vi "Parse-attributes.vi"(8 "error in (no error)":errorcluster, 10 "String in":string, 11 "Set in":refnum<class "Set.lvclass">) -> (0 "error out":errorcluster, 1 "Valid attributes?":bool, 2 "Remaining string":string, 3 "Set out":refnum<class "Set.lvclass">, 4 "Remaining content?":bool)   [LabVIEW 2013, in "HardwareCharacterization.lvlib" / "Set.lvclass"]
uses:
  Set.lvclass
  Attribute-XML/Attributes.ctl
  Attribute-XML/ID/Attribute-ID.ctl
  Attribute-XML/Attribute-XML.lvclass
  Attribute-XML/ID/FieldOffset/FieldOffset.lvclass
  Attribute-XML/ID/TransformEnable/TransformEnable.lvclass
  Attribute-XML/ID/Transform/Transform.lvclass
  Attribute-XML/ID/Units/Units.lvclass
  Attribute-XML/ID/XYCalFactor/XYCalFactor.lvclass
  Attribute-XML/ID/EnableLaser/EnableLaser.lvclass
  Attribute-XML/ID/JumpDelay/JumpDelay.lvclass
  Attribute-XML/ID/MarkDelay/MarkDelay.lvclass
  Attribute-XML/ID/PolyDelay/PolyDelay.lvclass
  Attribute-XML/ID/LaserOnDelay/LaserOnDelay.lvclass
  Attribute-XML/ID/LaserOffDelay/LaserOffDelay.lvclass
  Attribute-XML/ID/JumpSpeed/JumpSpeed.lvclass
  Attribute-XML/ID/MarkSpeed/MarkSpeed.lvclass
  Attribute-XML/ID/LaserPower/LaserPower.lvclass
  Attribute-XML/ID/Offset/Offset.lvclass
  Element-XML.lvclass/Element-XML.ctl
  Write Attributes.vi
  Attribute-XML/ID/ID.lvclass
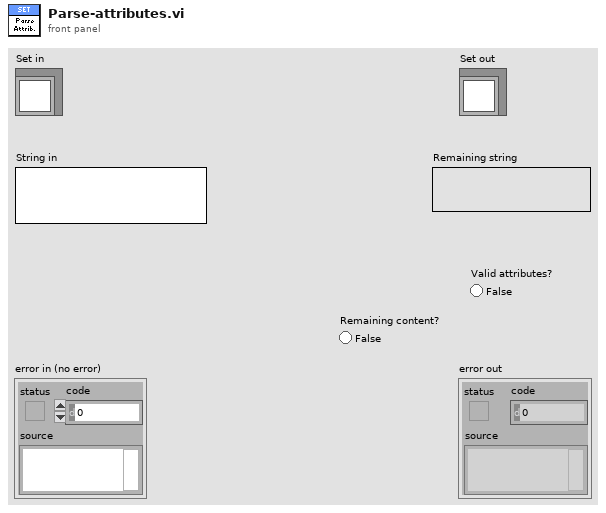
[diagram p1: front panel]
types:
  T1 = typedef "HardwareCharacterization.lvlib/ID.lvclass/Attribute-ID.ctl" = enum16{"FieldOffset", "TransformEnable", "Transform", "Units", "XYCalFactor", "EnableLaser", "JumpDelay", "MarkDelay", "PolyDelay", "LaserOnDelay", "LaserOffDelay", "JumpSpeed", "MarkSpeed", "LaserPowerDelay", "LaserEnableDelay", "LaserPower", "Offset"}
  T2 = typedef "HardwareCharacterization.lvlib/Attribute-XML.lvclass/Attributes.ctl" = enum16{"id"}
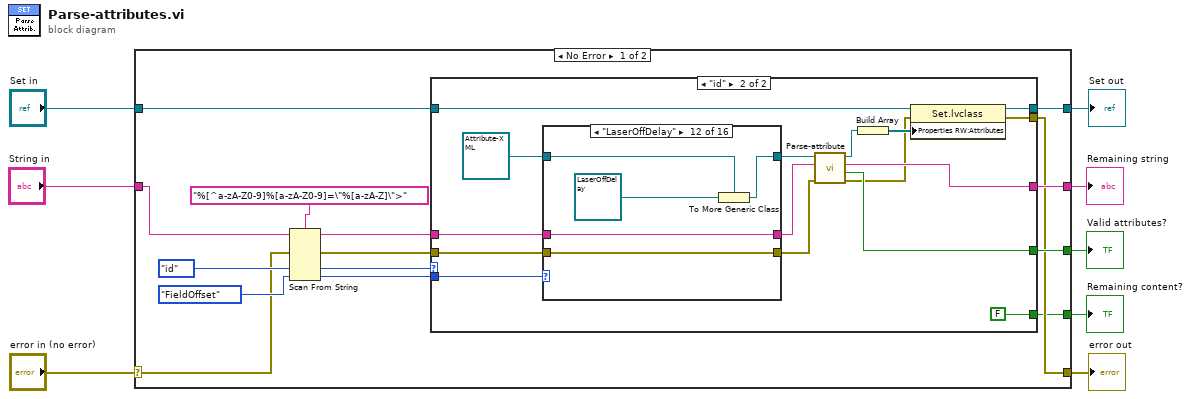
[diagram p0: block diagram]
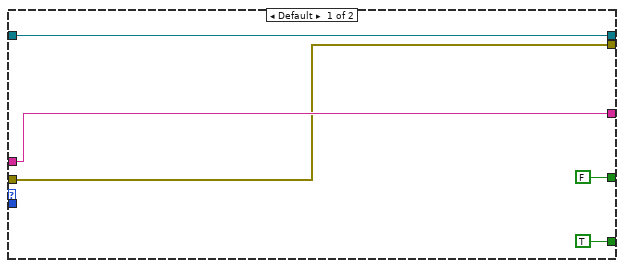
[diagram p2: hidden frame]
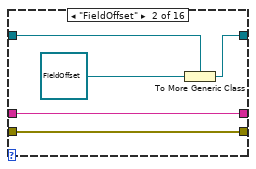
[diagram p4: hidden frame]
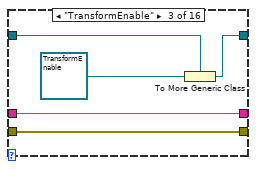
[diagram p5: hidden frame]
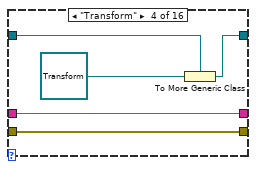
[diagram p6: hidden frame]
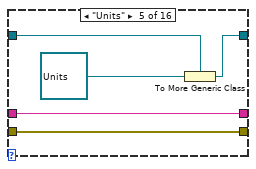
[diagram p7: hidden frame]
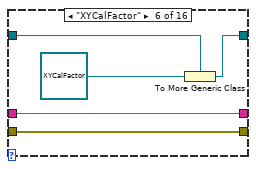
[diagram p8: hidden frame]
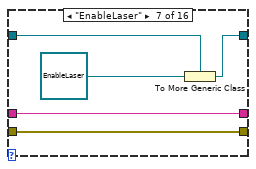
[diagram p9: hidden frame]
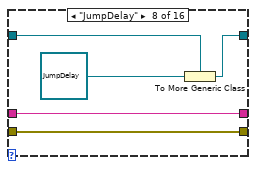
[diagram p10: hidden frame]
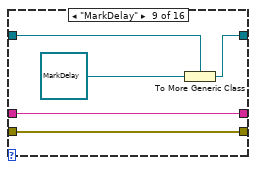
[diagram p11: hidden frame]
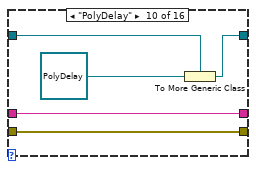
[diagram p12: hidden frame]
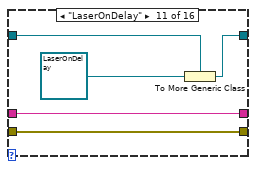
[diagram p13: hidden frame]
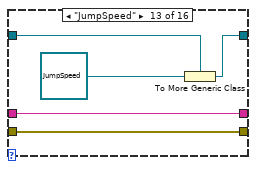
[diagram p14: hidden frame]
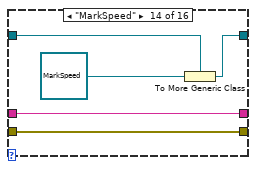
[diagram p15: hidden frame]
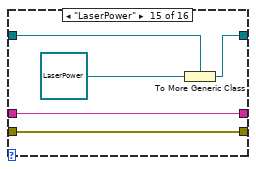
[diagram p16: hidden frame]
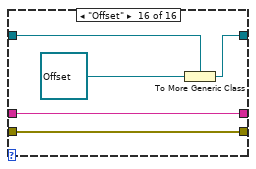
[diagram p17: hidden frame]
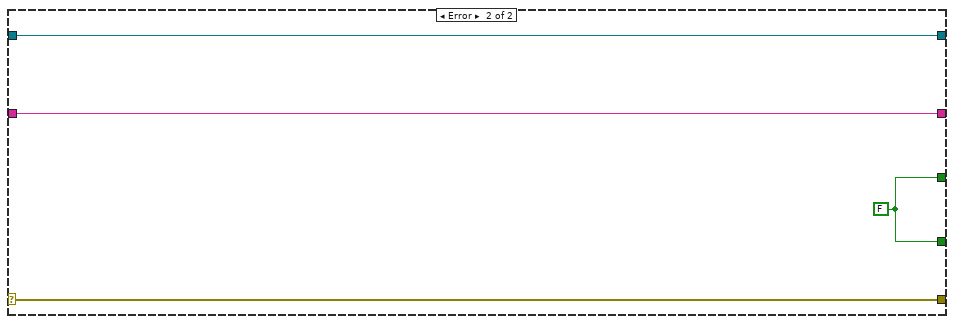
[diagram p18: hidden frame]
diagram:
  n1 = case shown="No Error" "error in (no error)" {
    selector: "error in (no error)" -> [w17 w126]
    tunnel: [w11 w126] -> w7
    tunnel: [w15 w125] -> w5
    tunnel: "Set in" -> [w14 w125]
    tunnel: "String in" -> [w16 w124]
    tunnel: [w13 w124] -> w3
    tunnel: [w12 w123] -> w2
    tunnel: [w9 w123] -> w1
    frame No Error {
      n2 = Scan From String(format string="%[^a-zA-Z0-9]%[a-zA-Z0-9]=\"%[a-zA-Z]\">", input string=w16, error in=w17, default 2=Attributes."id" ("Attribute"), default 3=Attribute-ID."FieldOffset" ("ID-attribute")) -> (remaining string=w20:string, error out=w22:errorcluster, output 2=w10:T2, output 3=w21:T1)  [unwired: 3 in, 1 out]
      n3 = case shown="\"id\"" w10 {
        tunnel: w22 -> [w26 w44]
        tunnel: w21 -> [_ w43]
        tunnel: w20 -> [w27 w42]
        tunnel: [w28 w41] -> w15
        tunnel: w14 -> [w28 w40]
        tunnel: [w27 w34] -> w13
        tunnel: [FALSE ("Valid attribute?") w32] -> w12
        tunnel: [w26 w30] -> w11
        tunnel: [TRUE FALSE] -> w9
        frame Default {
        }
        frame "id" {
          n4 = case shown="\"LaserOffDelay\"" w43 {
            tunnel: refnum<class "Attribute-XML.lvclass"> refnum ("Attribute-XML.lvclass") -> [w47 w51 w56 w61 w66 w71 w76 w81 w86 w91 w96 w101 w106 w111 w116 w121]
            tunnel: w44 -> [w46 w50 w55 w60 w65 w70 w75 w80 w85 w90 w95 w100 w105 w110 w115 w120]
            tunnel: [w47 w52 w57 w62 w67 w72 w77 w82 w87 w92 w97 w102 w107 w112 w117 w122] -> w37
            tunnel: [w46 w50 w55 w60 w65 w70 w75 w80 w85 w90 w95 w100 w105 w110 w115 w120] -> w35
            tunnel: w42 -> [w45 w49 w54 w59 w64 w69 w74 w79 w84 w89 w94 w99 w104 w109 w114 w119]
            tunnel: [w45 w49 w54 w59 w64 w69 w74 w79 w84 w89 w94 w99 w104 w109 w114 w119] -> w33
            frame Default {
            }
            frame "FieldOffset" {
              n5 = To More Generic Class(target class=w51, reference=refnum<class "FieldOffset.lvclass"> refnum ("FieldOffset.lvclass")) -> (generic class reference=w52:refnum<class "Attribute-XML.lvclass">)
            }
            frame "TransformEnable" {
              n6 = To More Generic Class(target class=w56, reference=refnum<class "TransformEnable.lvclass"> refnum ("TransformEnable.lvclass")) -> (generic class reference=w57:refnum<class "Attribute-XML.lvclass">)
            }
            frame "Transform" {
              n7 = To More Generic Class(target class=w61, reference=refnum<class "Transform.lvclass"> refnum ("Transform.lvclass")) -> (generic class reference=w62:refnum<class "Attribute-XML.lvclass">)
            }
            frame "Units" {
              n8 = To More Generic Class(target class=w66, reference=refnum<class "Units.lvclass"> refnum ("Units.lvclass")) -> (generic class reference=w67:refnum<class "Attribute-XML.lvclass">)
            }
            frame "XYCalFactor" {
              n9 = To More Generic Class(target class=w71, reference=refnum<class "XYCalFactor.lvclass"> refnum ("XYCalFactor.lvclass")) -> (generic class reference=w72:refnum<class "Attribute-XML.lvclass">)
            }
            frame "EnableLaser" {
              n10 = To More Generic Class(target class=w76, reference=refnum<class "EnableLaser.lvclass"> refnum ("EnableLaser.lvclass")) -> (generic class reference=w77:refnum<class "Attribute-XML.lvclass">)
            }
            frame "JumpDelay" {
              n11 = To More Generic Class(target class=w81, reference=refnum<class "JumpDelay.lvclass"> refnum ("JumpDelay.lvclass")) -> (generic class reference=w82:refnum<class "Attribute-XML.lvclass">)
            }
            frame "MarkDelay" {
              n12 = To More Generic Class(target class=w86, reference=refnum<class "MarkDelay.lvclass"> refnum ("MarkDelay.lvclass")) -> (generic class reference=w87:refnum<class "Attribute-XML.lvclass">)
            }
            frame "PolyDelay" {
              n13 = To More Generic Class(target class=w91, reference=refnum<class "PolyDelay.lvclass"> refnum ("PolyDelay.lvclass")) -> (generic class reference=w92:refnum<class "Attribute-XML.lvclass">)
            }
            frame "LaserOnDelay" {
              n14 = To More Generic Class(target class=w96, reference=refnum<class "LaserOnDelay.lvclass"> refnum ("LaserOnDelay.lvclass")) -> (generic class reference=w97:refnum<class "Attribute-XML.lvclass">)
            }
            frame "LaserOffDelay" {
              n15 = To More Generic Class(target class=w101, reference=refnum<class "LaserOffDelay.lvclass"> refnum ("LaserOffDelay.lvclass")) -> (generic class reference=w102:refnum<class "Attribute-XML.lvclass">)
            }
            frame "JumpSpeed" {
              n16 = To More Generic Class(target class=w106, reference=refnum<class "JumpSpeed.lvclass"> refnum ("JumpSpeed.lvclass")) -> (generic class reference=w107:refnum<class "Attribute-XML.lvclass">)
            }
            frame "MarkSpeed" {
              n17 = To More Generic Class(target class=w111, reference=refnum<class "MarkSpeed.lvclass"> refnum ("MarkSpeed.lvclass")) -> (generic class reference=w112:refnum<class "Attribute-XML.lvclass">)
            }
            frame "LaserPower" {
              n18 = To More Generic Class(target class=w116, reference=refnum<class "LaserPower.lvclass"> refnum ("LaserPower.lvclass")) -> (generic class reference=w117:refnum<class "Attribute-XML.lvclass">)
            }
            frame "Offset" {
              n19 = To More Generic Class(target class=w121, reference=refnum<class "Offset.lvclass"> refnum ("Offset.lvclass")) -> (generic class reference=w122:refnum<class "Attribute-XML.lvclass">)
            }
          }
          n20 = call-dynamic "Parse-attribute.vi"("error in (no error)"=w35, "String in"=w33, "Attribute-XML in"=w37) -> ("error out"=w31:errorcluster, "Valid attribute?"=w32:bool, "Remaining string"=w34:string, "Attribute-XML out"=w36:refnum<class "Attribute-XML.lvclass">)  [unwired: 5 in]
          n21 = Build Array(w36) -> (w38:refnum<class "Attribute-XML.lvclass">[])
          n22 = property class="Set.lvclass"(reference=w40, error in=w31, "Properties RW:Attributes"=w38) -> (reference out=w41:refnum<class "Set.lvclass">, error out=w30:errorcluster)
        }
      }
    }
    frame Error {
      w123 = FALSE
    }
  }
  "error out" <- w7
  "Set out" <- w5
  "Remaining string" <- w3
  "Valid attributes?" <- w2
  "Remaining content?" <- w1
